vi "AlliGator Add Image to Accumulated Image.vi"(6 "Weight (1)":dbl=1.0, 7 "Image Name":string, 8 "Error In":errorcluster, 9 "Dataset Index":i32, 10 "Accumulated Image Sum (in(":T1, 11 "New Image":T1) -> (0 "Error Out":errorcluster, 2 "Accumulated Image Sum (out)":T1)   [LabVIEW 2021, in "AlliGator Accumulated Dataset.lvlib"]
doc: "Adds a single <B>New Image</B> (gate image) to the <B>Accumulated Image Sum</B> (for that gate).\n\nIf the current <B>Dataset Index</B> is 0 (first dataset in the Series), the <B>Accumulated Image Sum</B> is cleared first."
uses:
  AlliGator Accumulated Dataset.lvlib
  <vilib>/vision/Image Controls.llb/IMAQ Image.ctl
  <vilib>/vision/NI_Vision_Development_Module.lvlib
  Image/Image.lvlib
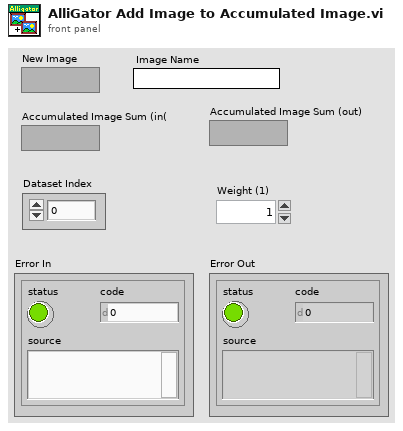
[diagram p1: front panel]
types:
  T1 = typedef "IMAQ Image.ctl" = refnum<image>
  T2 = typedef "Image Type" = u32
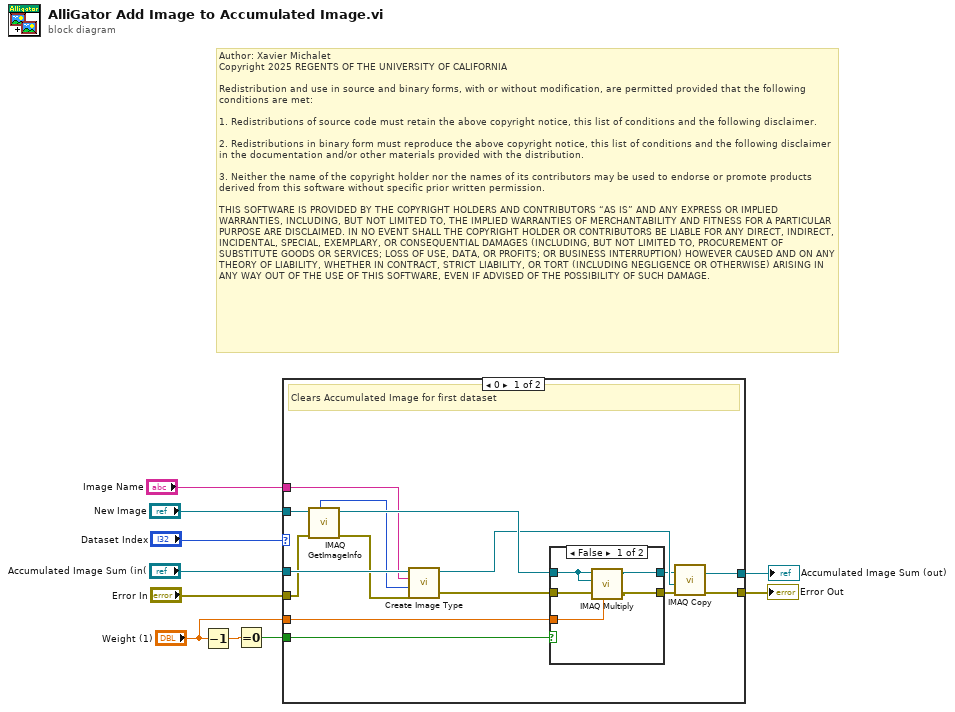
[diagram p0: block diagram]
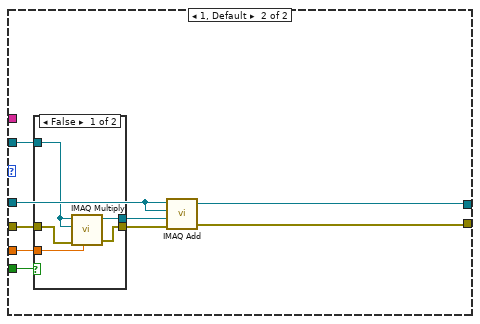
[diagram p3: hidden frame]
diagram:
  # "Author: Xavier Michalet\nCopyright 2025 REGENTS OF THE UNIVERSITY OF CALIFORNIA\n\nRedistribution and use in source and binary forms, with or without modification, are permitted provided that the following conditions are met:\n\n1. Redistributions of source code must retain the above copyright notice, this list of conditions and the following disclaimer.\n\n2. Redistributions in binary form must reproduce the above copyright notice, this list of conditions and the following disclaimer in the documentation and/or other materials provided with the distribution.\n\n3. Neither the name of the copyright holder nor the names of its contributors may be used to endorse or promote products derived from this software without specific prior written permission.\n\nTHIS SOFTWARE IS PROVIDED BY THE COPYRIGHT HOLDERS AND CONTRIBUTORS “AS IS” AND ANY EXPRESS OR IMPLIED WARRANTIES, INCLUDING, BUT NOT LIMITED TO, THE IMPLIED WARRANTIES OF MERCHANTABILITY AND FITNESS FOR A PARTICULAR PURPOSE ARE DISCLAIMED. IN NO EVENT SHALL THE COPYRIGHT HOLDER OR CONTRIBUTORS BE LIABLE FOR ANY DIRECT, INDIRECT, INCIDENTAL, SPECIAL, EXEMPLARY, OR CONSEQUENTIAL DAMAGES (INCLUDING, BUT NOT LIMITED TO, PROCUREMENT OF SUBSTITUTE GOODS OR SERVICES; LOSS OF USE, DATA, OR PROFITS; OR BUSINESS INTERRUPTION) HOWEVER CAUSED AND ON ANY THEORY OF LIABILITY, WHETHER IN CONTRACT, STRICT LIABILITY, OR TORT (INCLUDING NEGLIGENCE OR OTHERWISE) ARISING IN ANY WAY OUT OF THE USE OF THIS SOFTWARE, EVEN IF ADVISED OF THE POSSIBILITY OF SUCH DAMAGE."
  n1 = Decrement(x="Weight (1)") -> (x-1=w2:dbl)
  n2 = Equal To 0?(x=w2) -> (x = 0?=w1:bool)
  n3 = case shown="0" "Dataset Index" {
    tunnel: [w24 w40] -> w10
    tunnel: "New Image" -> [w20 w36]
    tunnel: "Image Name" -> [w11 _]
    tunnel: "Accumulated Image Sum (in(" -> [w23 w38]
    tunnel: "Error In" -> [w22 w33]
    tunnel: [w21 w39] -> w4
    tunnel: "Weight (1)" -> [w19 w34]
    tunnel: w1 -> [w16 w37]
    frame 0 {
      # "Clears Accumulated Image for first dataset"
      n4 = call "IMAQ GetImageInfo"("error in (no error)"=w22, "Image"=w20) -> ("error out"=w13:errorcluster, "Image Type"=w12:T2)  [unwired: 2 in, 6 out]
      n5 = call "Create Image Type.vi"("error in (no error)"=w13, "Image Type"=w12, "Image Name"=w11, "Refnum in"=w23) -> ("error out"=w18:errorcluster, "Refnum out"=w17:T1)  [unwired: 5 in, 1 out]
      n6 = case shown="False" w16 {
        tunnel: w20 -> [w29 w31]
        tunnel: [w27 w31] -> w15
        tunnel: w19 -> [w28 _]
        tunnel: w18 -> [w26 w30]
        tunnel: [w25 w30] -> w14
        frame False {
          n7 = call "IMAQ Multiply"("Image Src A"=w29, "Constant"=w28, "Image Dst"=w29, "error in (no error)"=w26) -> ("Image Dst Out"=w27:T1, "error out"=w25:errorcluster)  [unwired: 3 in]
        }
        frame True {
        }
      }
      n8 = call "IMAQ Copy"("error in (no error)"=w14, "Image Dst"=w17, "Image Src"=w15) -> ("error out"=w21:errorcluster, "Image Dst Out"=w24:T1)  [unwired: 3 in]
    }
    frame 1, Default {
      n9 = case shown="False" w37 {
        tunnel: w36 -> [w45 w47]
        tunnel: [w44 w47] -> w35
        tunnel: w34 -> [w43 _]
        tunnel: w33 -> [w42 w46]
        tunnel: [w41 w46] -> w32
        frame False {
          n10 = call "IMAQ Multiply"("Image Src A"=w45, "Constant"=w43, "Image Dst"=w45, "error in (no error)"=w42) -> ("Image Dst Out"=w44:T1, "error out"=w41:errorcluster)  [unwired: 3 in]
        }
        frame True {
        }
      }
      n11 = call "IMAQ Add"("Image Src A"=w38, "Image Dst"=w38, "Image Src B"=w35, "error in (no error)"=w32) -> ("Image Dst Out"=w40:T1, "error out"=w39:errorcluster)  [unwired: 3 in]
    }
  }
  "Accumulated Image Sum (out)" <- w10
  "Error Out" <- w4
